vi "GetTriOp.vi"(10 "Array":T3(array[cluster]), 11 "ModelName":string) -> (2 "Index":i32, 3 "TrianglesOut":T1[](array[typedef]))   [LabVIEW 2014]
uses:
  TypeDefs/TriangleFace.ctl
  TypeDefs/Point3D.ctl
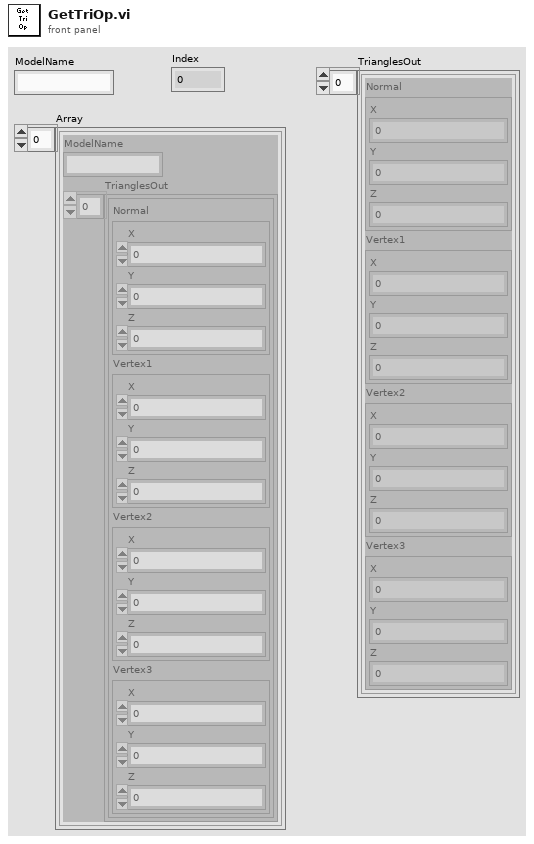
[diagram p1: front panel]
types:
  T1 = typedef "TriangleFace.ctl" = cluster{"Normal":T2, "Vertex1":T2, "Vertex2":T2, "Vertex3":T2}
  T2 = typedef "Point3D.ctl" = cluster{"X":sgl, "Y":sgl, "Z":sgl}
  T3 = cluster{"ModelName":string, "TrianglesOut":T1[]}[]
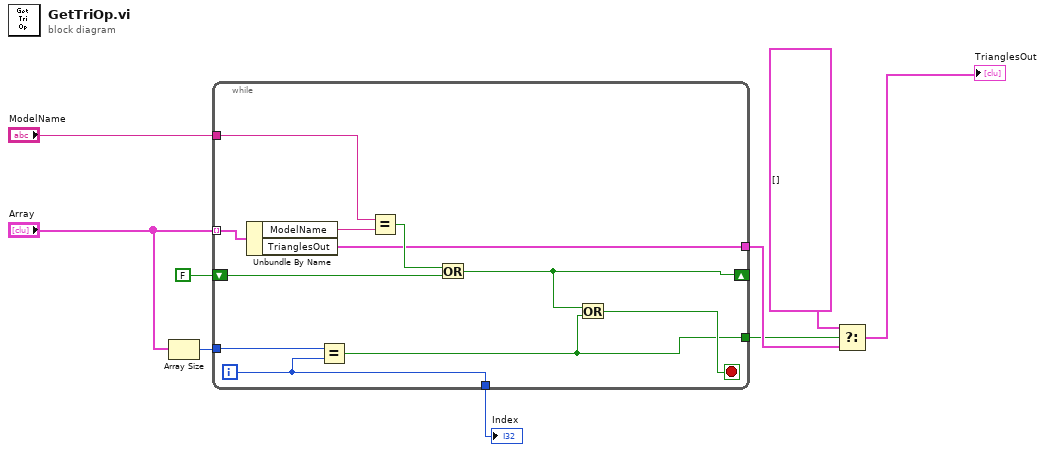
[diagram p0: block diagram]
diagram:
  n1 = Array Size(array="Array") -> (size(s)=w4:i32)
  n2 = while {
    tunnel: "ModelName" -> [w19]
    tunnel: "Array" -> [w20] mode=indexing
    shift-right: [w15] -> _
    shift-left: FALSE -> [w17]
    tunnel: w4 -> [w14]
    tunnel: [w12] -> w6
    tunnel: [w11] -> w5
    tunnel: [w10] -> w1
    i -> [w10]
    stop <- w13 stop-if-true
    n3 = Unbundle By Name(w20) -> ("ModelName"=w18:string, "TrianglesOut"=w12:T1[])
    n4 = Equal?(x=w14, y=w10) -> (x = y?=w11:bool)
    n5 = Equal?(x=w19, y=w18) -> (x = y?=w16:bool)
    n6 = Or(x=w16, y=w17) -> (x .or. y?=w15:bool)
    n7 = Or(x=w15, y=w11) -> (x .or. y?=w13:bool)
  }
  "Index" <- w1
  n8 = Select(t=T1[] [], s=w5, f=w6) -> (s? t:f=→"TrianglesOut":T1[])
